vi "Write Project Path.vi"(8 "error in (no error)":errorcluster, 10 "Project Path":path, 11 "Run UTF in":refnum<class "Run UTF.lvclass">) -> (0 "error out":errorcluster, 3 "Run UTF out":refnum<class "Run UTF.lvclass">)   [LabVIEW 2014, in "Run UTF.lvclass"]
uses:
  Run UTF.lvclass
  Run UTF.lvclass/Run UTF.ctl
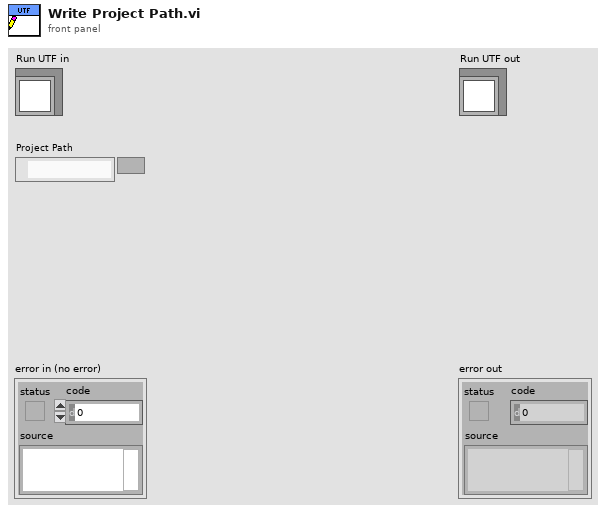
[diagram p1: front panel]
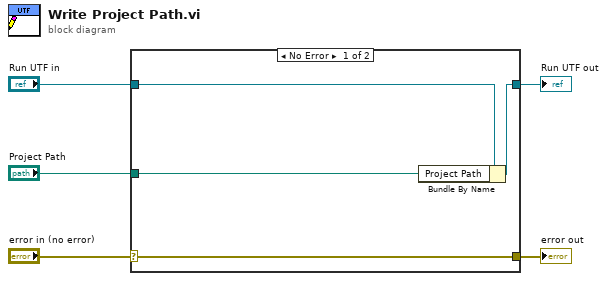
[diagram p0: block diagram]
diagram:
  n1 = case shown="No Error" "error in (no error)" {
    selector: "error in (no error)" -> [w9 w10]
    tunnel: [w9 w10] -> w4
    tunnel: [w7 w11] -> w2
    tunnel: "Run UTF in" -> [w8 w11]
    tunnel: "Project Path" -> [w6 _]
    frame No Error {
      n2 = Bundle By Name(cluster=w8, "Project Path"=w6) -> (w7:refnum<class "Run UTF.lvclass">)
    }
    frame Error {
    }
  }
  "error out" <- w4
  "Run UTF out" <- w2
